vi "Disconnect.vi"(8 "error in":errorcluster, 11 "Newport in":refnum<class "Newport.lvclass">) -> (0 "error out":errorcluster, 3 "Newport out":refnum<class "Newport.lvclass">)   [LabVIEW 2018, in "Newport.lvlib" / "Newport.lvclass"]
uses:
  Newport.lvclass
  Newport.XPS.CommandInterface
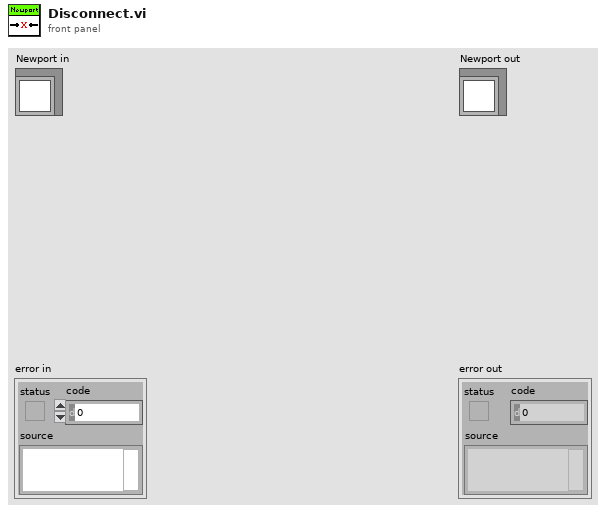
[diagram p1: front panel]
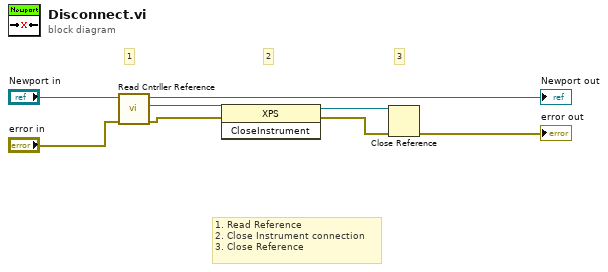
[diagram p0: block diagram]
diagram:
  # "1. Read Reference\n2. Close Instrument connection\n3. Close Reference"
  # "3"
  # "2"
  # "1"
  n1 = call-dynamic "Read Cntrller Reference.vi"("error in (no error)"="error in", "Newport in"="Newport in") -> ("error out"=w3:errorcluster, "Cntrller Reference"=w4:refnum<k24>, "Newport out"=→"Newport out":refnum<class "Newport.lvclass">)  [unwired: 7 in]
  n2 = invoke class="XPS" method="CloseInstrument"(reference=w4, error in=w3) -> (reference out=w5:refnum<k24>, error out=w6:errorcluster)  [unwired: 1 in, 1 out]
  n3 = Close Reference(reference=w5, error in (no error)=w6) -> (error out=→"error out":errorcluster)
